vi "UV_Head_CONN (SubVI).vi"(1 "Chn(coma deli)":string) -> (0 "Array":bool[](array[boolean]))   [LabVIEW 8.6]
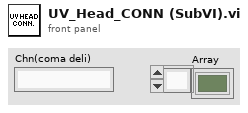
[diagram p1: front panel]
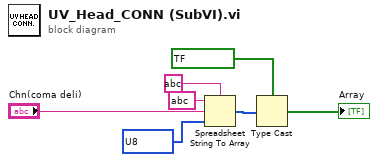
[diagram p0: block diagram]
diagram:
  n1 = Spreadsheet String To Array(delimiter (Tab)=string ?, format string=string ?, spreadsheet string="Chn(coma deli)", array type (2D Dbl)=u8[] ?) -> (array=w5:u8[])
  n2 = Type Cast(type=bool[] ?, x=w5) -> (*(type *) &x=→"Array":bool[])
